vi "Get User Interface VI.vi"(8 "error in (no error)":errorcluster, 11 "UDPlog Transfer Tx User Interface in":refnum<class "UDPlog Transfer Tx User Interface.lvclass">) -> (0 "error out":errorcluster, 2 "user interface vi":refnum<vi>, 3 "UDPlog Transfer Tx User Interface out":refnum<class "UDPlog Transfer Tx User Interface.lvclass">)   [LabVIEW 2023, in "UDPlog.lvlib" / "UDPlog Transfer Tx User Interface.lvclass"]
uses:
  UDPlog Transfer Tx User Interface.lvclass
  UDPlog Transfer Tx User Interface.lvclass/UDPlog Transfer Tx User Interface.ctl
  User Interface.vi
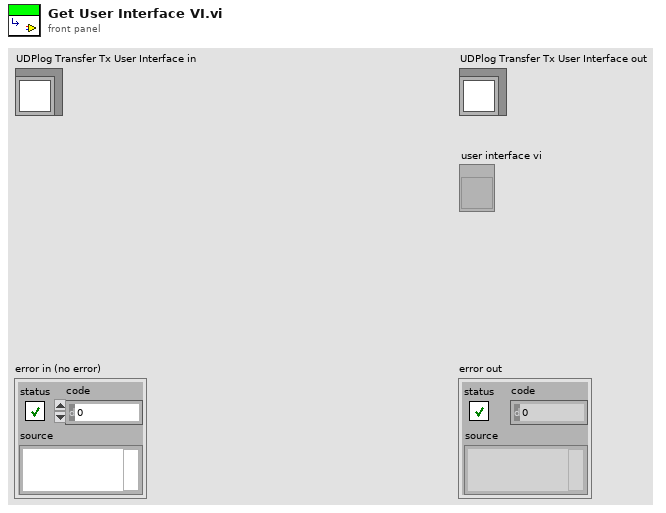
[diagram p1: front panel]
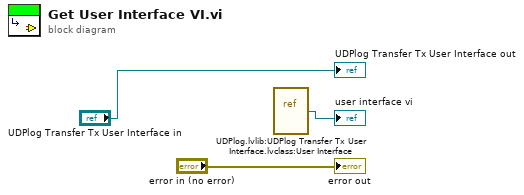
[diagram p0: block diagram]
diagram:
  n1 = vi-ref "UDPlog.lvlib:UDPlog Transfer Tx User Interface.lvclass:User Interface.vi"() -> (→"user interface vi":refnum<vi>)
  "error out" <- "error in (no error)"
  "UDPlog Transfer Tx User Interface out" <- "UDPlog Transfer Tx User Interface in"
